vi "Read Cycle period.vi"(8 "error in (no error)":errorcluster, 11 "Instrument Driver in":refnum<class "Instrument Driver.lvclass">) -> (0 "error out":errorcluster, 2 "Cycle period":dbl, 3 "Instrument Driver out":refnum<class "Instrument Driver.lvclass">)   [LabVIEW 2016, in "Instrument Driver.lvclass"]
uses:
  Instrument Driver.lvclass
  Instrument Driver.lvclass/Instrument Driver.ctl
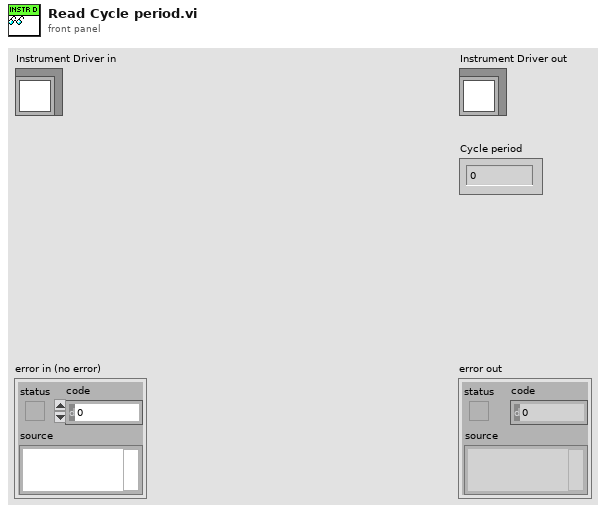
[diagram p1: front panel]
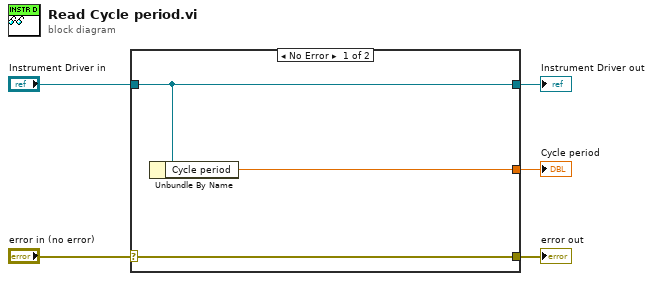
[diagram p0: block diagram]
diagram:
  n1 = case shown="No Error" "error in (no error)" {
    selector: "error in (no error)" -> [w8 w9]
    tunnel: [w8 w9] -> w4
    tunnel: [w7 w10] -> w2
    tunnel: "Instrument Driver in" -> [w7 w10]
    tunnel: [w6 _] -> w1
    frame No Error {
      n2 = Unbundle By Name(w7) -> ("Cycle period"=w6:dbl)
    }
    frame Error {
    }
  }
  "error out" <- w4
  "Instrument Driver out" <- w2
  "Cycle period" <- w1
